vi "Serialize as XML.vi"(8 "error in (no error)":errorcluster, 10 "Nesting Level":i32, 11 "Element in":refnum<class "Element.lvclass">) -> (0 "error out":errorcluster, 2 "XML Fragment":string, 3 "Element out":refnum<class "Element.lvclass">)   [LabVIEW 2026, in "VILab.lvlib" / "Element.lvclass"]
uses:
  Element.lvclass
  Element.lvclass/Element.ctl
  Attribute/Attribute.lvclass
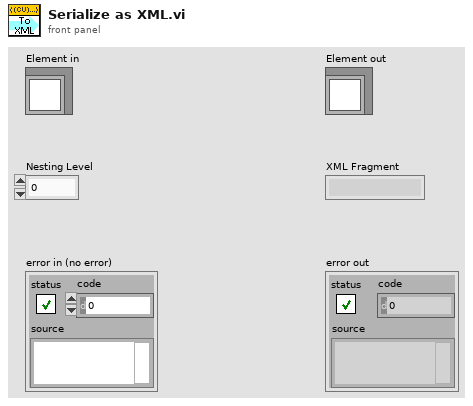
[diagram p1: front panel]
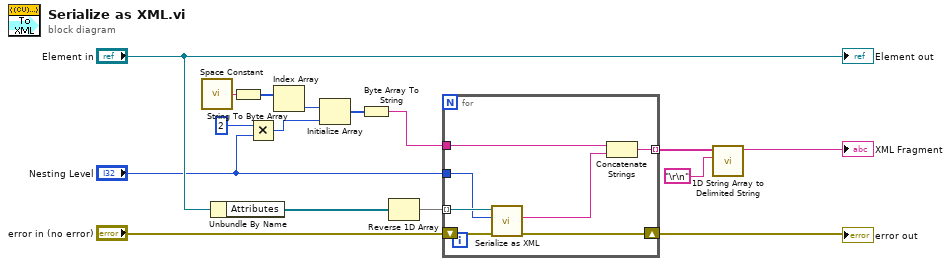
[diagram p0: block diagram]
diagram:
  n1 = call <vilib>:"Space Constant.vi"() -> ("String"=w7:string)
  n2 = Unbundle By Name("Element in") -> ("Attributes"=w13:refnum<class "Attribute.lvclass">[])
  n3 = String To Byte Array(string=w7) -> (unsigned byte array=w6:u8[])
  n4 = Multiply(x=2 ("y"), y="Nesting Level") -> (x*y=w3:i32)
  n5 = Index Array(array=w6) -> (element=w5:u8)  [unwired: 1 in]
  n6 = Initialize Array(w5, w3) -> (w4:u8[])
  n7 = Byte Array To String(unsigned byte array=w4) -> (string=w2:string)
  n8 = Reverse 1D Array(array=w13) -> (reversed array=w11:refnum<class "Attribute.lvclass">[])
  n9 = for {
    tunnel: w11 -> [w23] mode=indexing
    shift-right: [w21] -> w14
    shift-left: "error in (no error)" -> [w22]
    tunnel: [w18] -> w10 mode=indexing
    tunnel: "Nesting Level" -> [w19]
    tunnel: w2 -> [w17]
    n10 = call-dynamic "Serialize as XML.vi"("error in (no error)"=w22, "Nesting Level"=w19, "Attribute in"=w23) -> ("error out"=w21:errorcluster, "XML Fragment"=w20:string)  [unwired: 6 in, 1 out]
    n11 = Concatenate Strings(w17, w20) -> (w18:string)
  }
  "error out" <- w14
  n12 = call <vilib>:"1D String Array to Delimited String.vi"("delimiter"="\r\n", "string array"=w10) -> ("delimited string"=→"XML Fragment":string)  [unwired: 9 in]
  "Element out" <- "Element in"
